vi "Encrypt Decrypt Main Unitest.vi"(8 "error in (no error)":errorcluster, 9 "Process":enum16{"Decrypt", "Encrypt"}(ring), 11 "Input":string) -> (0 "error out":errorcluster, 3 "Output":string)   [LabVIEW 2025]
uses:
  <vilib>/Utility/error.llb/whitespace.ctl
  <vilib>/Utility/error.llb/Trim Whitespace One-Sided.vi
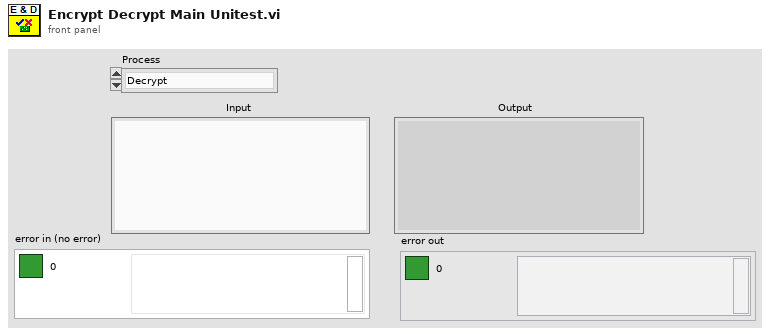
[diagram p1: front panel]
types:
  T1 = typedef "whitespace.ctl" = u16
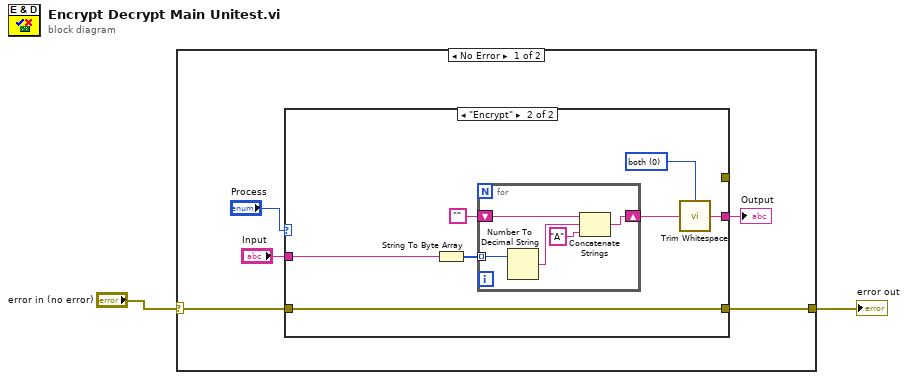
[diagram p0: block diagram]
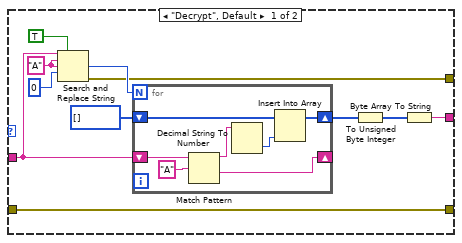
[diagram p2: hidden frame]
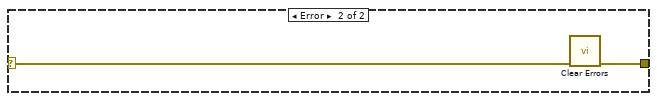
[diagram p3: hidden frame]
diagram:
  n1 = case shown="No Error" "error in (no error)" {
    selector: "error in (no error)" -> [w3 w39]
    tunnel: [w4 w38] -> w1
    frame No Error {
      n2 = case shown="\"Encrypt\"" "Process" {
        tunnel: "Input" -> [w17 w32]
        tunnel: [w11 w27] -> w5
        tunnel: [w9 _] -> _
        tunnel: [w8 w26] -> w4
        tunnel: w3 -> [w8 w26]
        frame "Decrypt", Default {
          w16 = "A" ("search string")
          n3 = Search and Replace String(replace all?=TRUE ("replace all? (F)"), input string=w17, search string=w16, replace string=w16, offset=0 ("offset (0)")) -> (number of replacements=w14:i32, error out=w9:errorcluster)  [unwired: 3 in, 2 out]
          n4 = for {
            N: w14 -> [_]
            shift-right: [w24] -> _
            shift-left: w17 -> [w25]
            shift-right: [w19] -> w12
            shift-left: i32[] [] -> [w21]
            n5 = Match Pattern(string=w25, regular expression="A") -> (before substring=w22:string, after substring=w24:string)  [unwired: 1 in, 2 out]
            n6 = Decimal String To Number(string=w22) -> (number=w20:i32)  [unwired: 2 in, 1 out]
            n7 = Insert Into Array(array=w21, new element=w20) -> (w19:i32[])  [unwired: 1 in]
          }
          n8 = To Unsigned Byte Integer(number=w12) -> (unsigned 8bit integer=w10:u8[])
          n9 = Byte Array To String(unsigned byte array=w10) -> (string=w11:string)
        }
        frame "Encrypt" {
          w28 = T1 0 items=["both", "start of string", "end of string"] ("location (both)")
          n10 = String To Byte Array(string=w32) -> (unsigned byte array=w31:u8[])
          n11 = for {
            tunnel: w31 -> [w35] mode=indexing
            shift-right: [w33] -> w29
            shift-left: "" -> [w37]
            n12 = Number To Decimal String(number=w35) -> (decimal integer string=w36:string)  [unwired: 1 in]
            n13 = Concatenate Strings(w37, w36, "A" ("string")) -> (w33:string)
          }
          n14 = call <vilib>:"Trim Whitespace.vi"("string"=w29, "location (both)"=w28) -> ("trimmed string"=w27:string)
        }
      }
      "Output" <- w5
    }
    frame Error {
      n15 = call <vilib>:"Clear Errors.vi"("error in (no error)"=w39) -> ("error out"=w38:errorcluster)  [unwired: 5 in, 1 out]
    }
  }
  "error out" <- w1
